vi "About.vi"() -> ()   [LabVIEW 2022 SP3]
panel:
  in  "OK":bool
  # "911X Power Supply Operating Software"
  # "Version    1.0.0"
  # "Copyright (c) 2020-2021\n\nB&K Precision Corporation. All rights reserved."
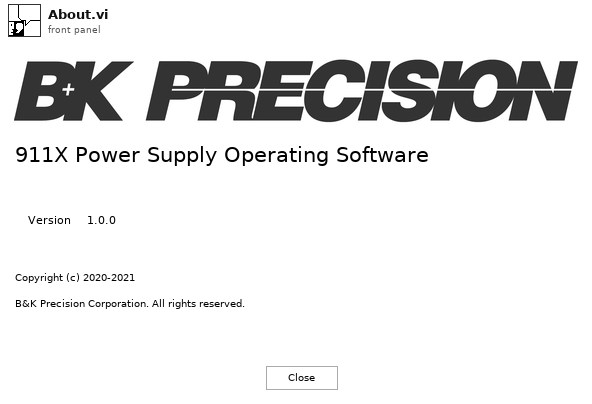
[diagram p1: front panel]
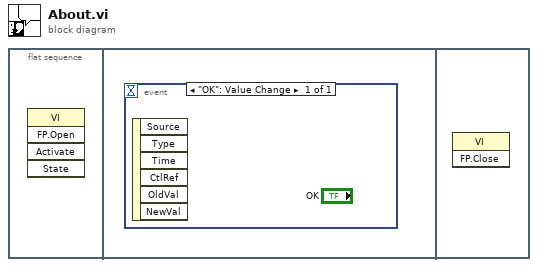
[diagram p0: block diagram]
diagram:
  n1 = flat-sequence {
    frame #0 {
      n2 = invoke class="VI" method="FP.Open"() -> ()  [unwired: 5 in, 5 out]
    }
    frame #1 {
      n3 = event shown="[0] \"OK\": Value Change" {
        selector: _ -> [_]
        dyn-events: _ -> [_]
        timeout: _ -> [_]
        event "OK": Value Change {
          n4 = event-data() -> ()  [unwired: 1 in, 6 out]
        }
      }
    }
    frame #2 {
      n5 = invoke class="VI" method="FP.Close"() -> ()  [unwired: 3 in, 3 out]
    }
  }
